vi "createCommand.vi"(8 "error in (no error)":errorcluster, 10 "Command":T1, 11 "CommandFactory in":refnum<class "CommandFactory.lvclass">) -> (0 "error out":errorcluster, 2 "command":refnum<class "Command.lvclass">, 3 "CommandFactory out":refnum<class "CommandFactory.lvclass">)   [LabVIEW 2015, in "CommandFactory.lvclass"]
uses:
  CommandFactory.lvclass
  Command/Command.lvclass
  Typedefs/CommandSelector.ctl
  Commands/ClearError/ClearError.lvclass
  Commands/Exit/Exit.lvclass
  Commands/StandBy/StandBy.lvclass
  Commands/Start/Start.lvclass
  Commands/Update/Update.lvclass
  Commands/StartTestScenarioCommand/StartTestScenarioCommand.lvclass
  Typedefs/ILCBTTypedefs.lvlib
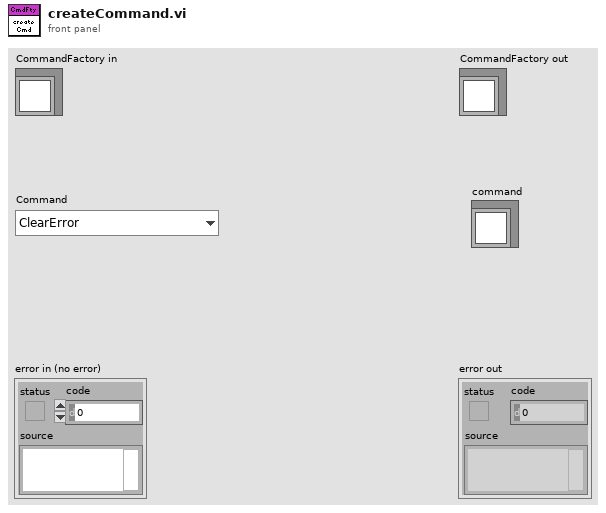
[diagram p1: front panel]
types:
  T1 = typedef "ILCBTTypedefs.lvlib/CommandSelector.ctl" = enum16{"ClearError", "Exit", "StandBy", "Start", "Update", "StartTestScenario"}
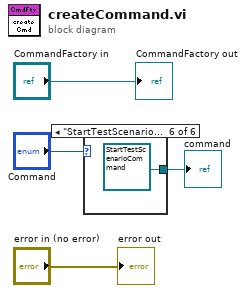
[diagram p0: block diagram]
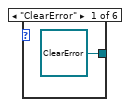
[diagram p2: hidden frame]
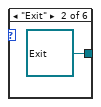
[diagram p3: hidden frame]
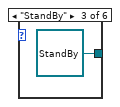
[diagram p4: hidden frame]
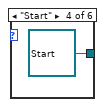
[diagram p5: hidden frame]
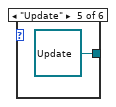
[diagram p6: hidden frame]
diagram:
  n1 = case shown="\"StartTestScenario\"" "Command" {
    tunnel: [refnum<class "ClearError.lvclass"> refnum ("ClearError.lvclass") refnum<class "Exit.lvclass"> refnum ("Exit.lvclass") refnum<class "StandBy.lvclass"> refnum ("StandBy.lvclass") refnum<class "Start.lvclass"> refnum ("Start.lvclass") refnum<class "Update.lvclass"> refnum ("Update.lvclass") refnum<class "StartTestScenarioCommand.lvclass"> refnum ("StartTestScenarioCommand.lvclass")] -> w2
    frame "ClearError" {
    }
    frame "Exit" {
    }
    frame "StandBy" {
    }
    frame "Start" {
    }
    frame "Update" {
    }
    frame "StartTestScenario" {
    }
  }
  "command" <- w2
  "error out" <- "error in (no error)"
  "CommandFactory out" <- "CommandFactory in"
